vi "3. Термометр.vi"() -> ()   [LabVIEW 2020]
panel:
  out "Waveform Chart":dbl(graph)
  in  "остановка":bool
  out "Текущее значение температуры \nв градусах Реамюра, R":dbl format="%#.1f"
  out "Текущее значение температуры\nв градусах Фаренгейта, F":dbl format="%#.1f"
  out "Температура в градусах Реамюра, R":dbl(slide) scale=0.0..21.0
  out "Температура в градусах Фаренгейта, F":dbl(slide) scale=0.0..78.0
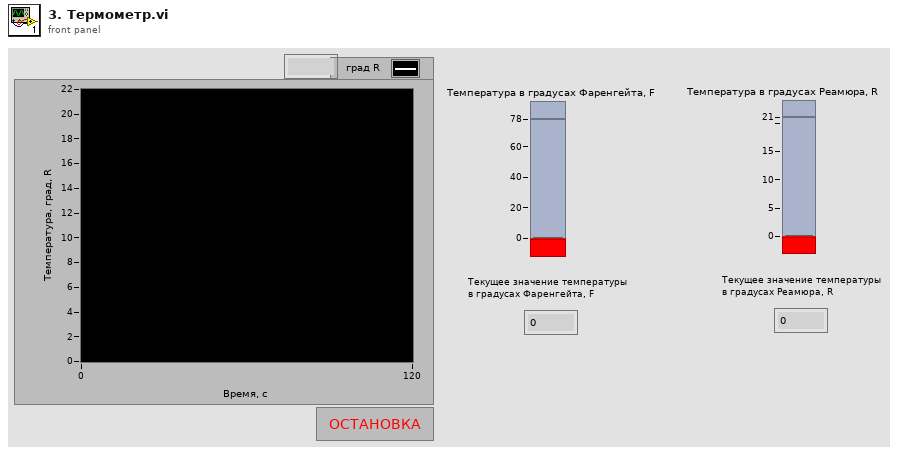
[diagram p1: front panel]
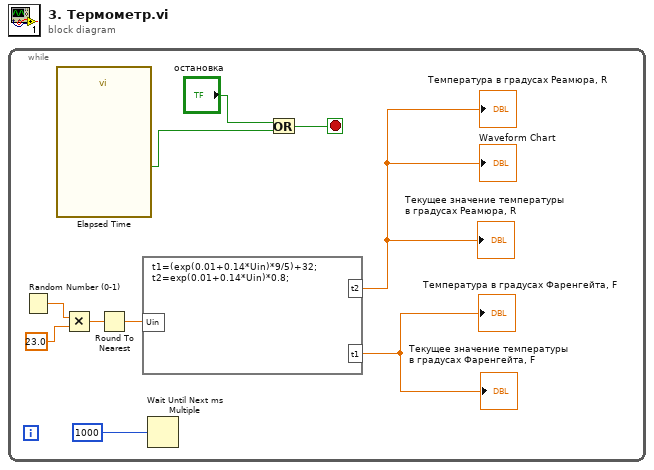
[diagram p0: block diagram]
diagram:
  n1 = while {
    stop <- w6 stop-if-true
    n2 = Random Number (0-1)() -> (number: 0 to 1=w9:dbl)
    n3 = call "Elapsed Time"() -> ("Time has Elapsed"=w4:bool)  [unwired: 12 in, 7 out]
    n4 = Multiply(x=w9, y=23.0) -> (x*y=w10:dbl)
    n5 = Round To Nearest(number=w10) -> (nearest integer value=w5:dbl)
    n6 = formula code="t1=(exp(0.01+0.14*Uin)*9/5)+32;\nt2=exp(0.01+0.14*Uin)*0.8;"("Uin"=w5) -> ("t1"=→"Температура в градусах Фаренгейта, F" →"Текущее значение температуры\nв градусах Фаренгейта, F":dbl, "t2"=→"Температура в градусах Реамюра, R" →"Текущее значение температуры \nв градусах Реамюра, R" →"Waveform Chart":dbl)
    n7 = Wait Until Next ms Multiple(millisecond multiple=u32 1000 ("millisecond timer value")) -> ()  [unwired: 1 out]
    n8 = Or(x="остановка", y=w4) -> (x .or. y?=w6:bool)
  }
